vi "Double2Float.vi"(7 "float":dbl) -> (8 "string":string)   [LabVIEW 2022 SP3]
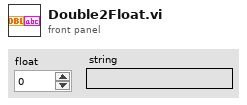
[diagram p1: front panel]
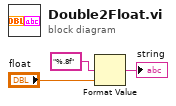
[diagram p0: block diagram]
diagram:
  n1 = Format Value(format string="%.8f", value (0)="float") -> (output string=→"string":string)  [unwired: 1 in]
